vi "rsidr_core_global.vi"() -> ()   [LabVIEW 2020, in "Rohde&Schwarz RTx Oscilloscopes.lvlib"] (continued)
Options"="", "Flags"=0, "Help"="Searches for a subsystem bit of a status word.\n01X-string\n\nAvailable Repeated Capabilities:\nNone\n\nRemote-control command(s):\nSEARch:PROTocol:MILStd:STATus:SUBSystem"}, {"Level"=4, "Class Only"=FALSE, "Identifier"="RSRTX_ATTR_MILSTD_SEARCH_TERMINAL_BIT_STATUS", "Descriptive Name"="MILSTD Search Terminal Bit Status", "Data Type"=0, "Command"="SEAR:PROT:MILS:STAT:TERM", "Access"=2, "Range Table"="rsrtx_rngStatus", "Read Callback"="", "Write Callback"="", "Supported Models"="RTM|RTA", "Instrument Options"="", "Flags"=0, "Help"="Searches for a terminal bit of a status word.\n01X-string\n\nAvailable Repeated Capabilities:\nNone\n\nRemote-control command(s):\nSEARch:PROTocol:MILStd:STATus:TERMinal"}, {"Level"=3, "Class Only"=TRUE, "Identifier"="", "Descriptive Name"="Data", "Data Type"=0, "Command"="", "Access"=0, "Range Table"="", "Read Callback"="", "Write Callback"="", "Supported Models"="", "Instrument Options"="", "Flags"=0, "Help"="Searches for a data, that is specified."}, {"Level"=4, "Class Only"=FALSE, "Identifier"="RSRTX_ATTR_MILSTD_SEARCH_DATA_CONDITION", "Descriptive Name"="MILSTD Search Data Condition", "Data Type"=0, "Command"="SEAR:PROT:MILS:DATA:COND", "Access"=2, "Range Table"="rsrtx_rngMILSTDCondition", "Read Callback"="", "Write Callback"="", "Supported Models"="RTM|RTA", "Instrument Options"="", "Flags"=0, "Help"="For a data word, searches for a comparison condition.\n\nAvailable Repeated Capabilities:\nNone\n\nRemote-control command(s):\nSEARch:PROTocol:MILStd:DATA:CONDition"}, {"Level"=4, "Class Only"=FALSE, "Identifier"="RSRTX_ATTR_MILSTD_SEARCH_DATA_MINIMUM", "Descriptive Name"="MILSTD Search Data Minimum", "Data Type"=2, "Command"="SEAR:PROT:MILS:DATA:MIN", "Access"=2, "Range Table"="", "Read Callback"="", "Write Callback"="", "Supported Models"="RTM|RTA", "Instrument Options"="", "Flags"=0, "Help"="For a data word, searches for a minimum value.\n01X-string\n\nAvailable Repeated Capabilities:\nNone\n\nRemote-control command(s):\nSEARch:PROTocol:MILStd:DATA:MINimum"}, {"Level"=4, "Class Only"=FALSE, "Identifier"="RSRTX_ATTR_MILSTD_SEARCH_DATA_MAXIMUM", "Descriptive Name"="MILSTD Search Data Maximum", "Data Type"=2, "Command"="SEAR:PROT:MILS:DATA:MAX", "Access"=2, "Range Table"="", "Read Callback"="", "Write Callback"="", "Supported Models"="RTM|RTA", "Instrument Options"="", "Flags"=0, "Help"="For a data word, searches for a maximum value.\n01X-string\n\nAvailable Repeated Capabilities:\nNone\n\nRemote-control command(s):\nSEARch:PROTocol:MILStd:DATA:MAXimum"}, {"Level"=4, "Class Only"=FALSE, "Identifier"="RSRTX_ATTR_MILSTD_SEARCH_DATA_OFFSET", "Descriptive Name"="MILSTD Search Data Offset", "Data Type"=0, "Command"="SEAR:PROT:MILS:DATA:OFFS", "Access"=2, "Range Table"="", "Read Callback"="", "Write Callback"="", "Supported Models"="RTM|RTA", "Instrument Options"="", "Flags"=0, "Help"="For a data word, searches for a data offset.\n\nAvailable Repeated Capabilities:\nNone\n\nRemote-control command(s):\nSEARch:PROTocol:MILStd:DATA:OFFSet"}, {"Level"=4, "Class Only"=FALSE, "Identifier"="RSRTX_ATTR_MILSTD_SEARCH_DATA_OFFSET_WORDS", "Descriptive Name"="MILSTD Search Data Offset Words", "Data Type"=0, "Command"="SEAR:PROT:MILS:DATA:WORD", "Access"=2, "Range Table"="", "Read Callback"="", "Write Callback"="", "Supported Models"="RTM|RTA", "Instrument Options"="", "Flags"=0, "Help"="For a data word, searches for a number of words.\n\nAvailable Repeated Capabilities:\nNone\n\nRemote-control command(s):\nSEARch:PROTocol:MILStd:DATA:WORDs"}, {"Level"=2, "Class Only"=TRUE, "Identifier"="", "Descriptive Name"="ARINC 429", "Data Type"=0, "Command"="", "Access"=0, "Range Table"="", "Read Callback"="", "Write Callback"="", "Supported Models"="", "Instrument Options"="", "Flags"=0, "Help"="Configures ARINC 429 search settings."}, {"Level"=3, "Class Only"=FALSE, "Identifier"="RSRTX_ATTR_PROTOCOL_ARINC429_SEARCH_TYPE", "Descriptive Name"="Protocol ARINC429 Search Type", "Data Type"=0, "Command"="SEAR:PROT:ARIN:COND", "Access"=2, "Range Table"="rsrtx_rngARINC429Type", "Read Callback"="", "Write Callback"="", "Supported Models"="RTM|RTA", "Instrument Options"="", "Flags"=0, "Help"="Sets the event or combination of events to be searched for. Depending on the selected event, further settings are required.\n\nAvailable Repeated Capabilities:\nNone\n\nRemote-control command(s):\nSEARch:PROTocol:ARINc:CONDition"}, {"Level"=3, "Class Only"=FALSE, "Identifier"="RSRTX_ATTR_PROTOCOL_ARINC429_SEARCH_WORD_TYPE", "Descriptive Name"="Protocol ARINC429 Search Word Type", "Data Type"=0, "Command"="SEAR:PROT:ARIN:WORD", "Access"=2, "Range Table"="rsrtx_rngARINC429WordType", "Read Callback"="", "Write Callback"="", "Supported Models"="RTM|RTA", "Instrument Options"="", "Flags"=0, "Help"="Selects the word type to be searched for.\n\nAvailable Repeated Capabilities:\nNone\n\nRemote-control command(s):\nSEARch:PROTocol:ARINc:WORD[:TYPE]"}, {"Level"=3, "Class Only"=FALSE, "Identifier"="RSRTX_ATTR_PROTOCOL_ARINC429_SEARCH_ERROR", "Descriptive Name"="Protocol ARINC429 Search Error", "Data Type"=0, "Command"="SEAR:PROT:ARIN:ERR", "Access"=2, "Range Table"="rsrtx_rngARINC429Error", "Read Callback"="", "Write Callback"="", "Supported Models"="RTM|RTA", "Instrument Options"="", "Flags"=0, "Help"="Searches for an error condition.\n\nAvailable Repeated Capabilities:\nNone\n\nRemote-control command(s):\nSEARch:PROTocol:ARINc:ERRor"}, {"Level"=3, "Class Only"=TRUE, "Identifier"="", "Descriptive Name"="Label Data", "Data Type"=0, "Command"="", "Access"=0, "Range Table"="", "Read Callback"="", "Write Callback"="", "Supported Models"="", "Instrument Options"="", "Flags"=0, "Help"="Configures ARINC 429 search label+data settings."}, {"Level"=4, "Class Only"=FALSE, "Identifier"="RSRTX_ATTR_PROTOCOL_ARINC429_SEARCH_LABEL_PATTERN_CONDITION", "Descriptive Name"="Protocol ARINC429 Search Label Pattern Condition", "Data Type"=0, "Command"="SEAR:PROT:ARIN:LAB:COND", "Access"=2, "Range Table"="rsrtx_rngProtocolARINC429Operator", "Read Callback"="", "Write Callback"="", "Supported Models"="RTM|RTA", "Instrument Options"="", "Flags"=0, "Help"="Sets the comparison condition for label: If the pattern contains at least one X (don&apos;t care), you can trigger on values equal or not equal to the specified value. If the pattern contains only 0 and 1, you can also trigger on a range greater than or lower than the specified value.\n\nAvailable Repeated Capabilities:\nNone\n\nRemote-control command(s):\nSEARch:PROTocol:ARINc:LABel:CONDition"}, {"Level"=4, "Class Only"=FALSE, "Identifier"="RSRTX_ATTR_PROTOCOL_ARINC429_SEARCH_LABEL_PATTERN_MIN", "Descriptive Name"="Protocol ARINC429 Search Label Pattern Min", "Data Type"=2, "Command"="SEAR:PROT:ARIN:LAB:MIN", "Access"=2, "Range Table"="", "Read Callback"="", "Write Callback"="", "Supported Models"="RTM|RTA", "Instrument Options"="", "Flags"=0, "Help"="Searches for a minimum value of the label.\n\nAvailable Repeated Capabilities:\nNone\n\nRemote-control command(s):\nSEARch:PROTocol:ARINc:LABel:MINimum"}, {"Level"=4, "Class Only"=FALSE, "Identifier"="RSRTX_ATTR_PROTOCOL_ARINC429_SEARCH_LABEL_PATTERN_MAX", "Descriptive Name"="Protocol ARINC429 Search Label Pattern Max", "Data Type"=2, "Command"="SEAR:PROT:ARIN:LAB:MAX", "Access"=2, "Range Table"="", "Read Callback"="", "Write Callback"="", "Supported Models"="RTM|RTA", "Instrument Options"="", "Flags"=0, "Help"="Searches for a maximum value of the label if Label Pattern Condition is set to InRange or OutOfRange.\n\nAvailable Repeated Capabilities:\nNone\n\nRemote-control command(s):\nSEARch:PROTocol:ARINc:LABel:MAXimum"}, {"Level"=4, "Class Only"=FALSE, "Identifier"="RSRTX_ATTR_PROTOCOL_ARINC429_SEARCH_DATA_PATTERN_CONDITION", "Descriptive Name"="Protocol ARINC429 Search Data Pattern Condition", "Data Type"=0, "Command"="SEAR:PROT:ARIN:DATA:COND", "Access"=2, "Range Table"="rsrtx_rngProtocolARINC429Operator", "Read Callback"="", "Write Callback"="", "Supported Models"="RTM|RTA", "Instrument Options"="", "Flags"=0, "Help"="Sets the comparison condition for datal: If the pattern contains at least one X (don&apos;t care), you can trigger on values equal or not equal to the specified value. If the pattern contains only 0 and 1, you can also trigger on a range greater than or lower than the specified value.\n\nAvailable Repeated Capabilities:\nNone\n\nRemote-control command(s):\nSEARch:PROTocol:ARINc:DATA:CONDition"}, {"Level"=4, "Class Only"=FALSE, "Identifier"="RSRTX_ATTR_PROTOCOL_ARINC429_SEARCH_DATA_PATTERN_MIN", "Descriptive Name"="Protocol ARINC429 Search Data Pattern Min", "Data Type"=2, "Command"="SEAR:PROT:ARIN:DATA:MIN", "Access"=2, "Range Table"="", "Read Callback"="", "Write Callback"="", "Supported Models"="RTM|RTA", "Instrument Options"="", "Flags"=0, "Help"="Searches for a minimum value of the data.\n\nAvailable Repeated Capabilities:\nNone\n\nRemote-control command(s):\nSEARch:PROTocol:ARINc:DATA:MINimum"}, {"Level"=4, "Class Only"=FALSE, "Identifier"="RSRTX_ATTR_PROTOCOL_ARINC429_SEARCH_DATA_PATTERN_MAX", "Descriptive Name"="Protocol ARINC429 Search Data Pattern Max", "Data Type"=2, "Command"="SEAR:PROT:ARIN:DATA:MAX", "Access"=2, "Range Table"="", "Read Callback"="", "Write Callback"="", "Supported Models"="RTM|RTA", "Instrument Options"="", "Flags"=0, "Help"="Searches for a maximum value of the data  if Data Pattern Condition is set to InRange or OutOfRange.\n\nAvailable Repeated Capabilities:\nNone\n\nRemote-control command(s):\nSEARch:PROTocol:ARINc:DATA:MAX"}, {"Level"=4, "Class Only"=FALSE, "Identifier"="RSRTX_ATTR_PROTOCOL_ARINC429_SEARCH_DATA_OFFSET", "Descriptive Name"="Protocol ARINC429 Search Data Offset", "Data Type"=0, "Command"="SEAR:PROT:ARIN:DATA:OFFS", "Access"=2, "Range Table"="", "Read Callback"="", "Write Callback"="", "Supported Models"="RTM|RTA", "Instrument Options"="", "Flags"=0, "Help"="Searches for specified data offset.\n\nAvailable Repeated Capabilities:\nNone\n\nRemote-control command(s):\nSEARch:PROTocol:ARINc:DATA:OFFSet"}, {"Level"=4, "Class Only"=FALSE, "Identifier"="RSRTX_ATTR_PROTOCOL_ARINC429_SEARCH_DATA_SIZE", "Descriptive Name"="Protocol ARINC429 Search Data Size", "Data Type"=0, "Command"="SEAR:PROT:ARIN:DATA:SIZE", "Access"=2, "Range Table"="", "Read Callback"="", "Write Callback"="", "Supported Models"="RTM|RTA", "Instrument Options"="", "Flags"=0, "Help"="Searches for specified data size.\n\nAvailable Repeated Capabilities:\nNone\n\nRemote-control command(s):\nSEARch:PROTocol:ARINc:DATA:SIZE"}, {"Level"=4, "Class Only"=FALSE, "Identifier"="RSRTX_ATTR_PROTOCOL_ARINC429_SEARCH_DATA_FORMAT", "Descriptive Name"="Protocol ARINC429 Search Data Format", "Data Type"=0, "Command"="SEAR:PROT:ARIN:FORM", "Access"=2, "Range Table"="rsrtx_rngProtocolARINC429DataFormat", "Read Callback"="", "Write Callback"="", "Supported Models"="RTM|RTA", "Instrument Options"="", "Flags"=0, "Help"="Searches for a data format.\n\nAvailable Repeated Capabilities:\nNone\n\nRemote-control command(s):\nSEARch:PROTocol:ARINc:FORMat"}, {"Level"=4, "Class Only"=FALSE, "Identifier"="RSRTX_ATTR_PROTOCOL_ARINC429_SEARCH_SDI", "Descriptive Name"="Protocol ARINC429 Search SDI", "Data Type"=0, "Command"="SEAR:PROT:ARIN:SDI", "Access"=2, "Range Table"="rsrtx_rngARINCSsmSdi", "Read Callback"="", "Write Callback"="", "Supported Models"="RTM|RTA", "Instrument Options"="", "Flags"=0, "Help"="Searches for the specified source/destination identifier (SDI) bits.\n\nAvailable Repeated Capabilities:\nNone\n\nRemote-control command(s):\nSEARch:PROTocol:ARINc:SDI"}, {"Level"=4, "Class Only"=FALSE, "Identifier"="RSRTX_ATTR_PROTOCOL_ARINC429_SEARCH_SSM", "Descriptive Name"="Protocol ARINC429 Search SSM", "Data Type"=0, "Command"="SEAR:PROT:ARIN:SSM", "Access"=2, "Range Table"="rsrtx_rngARINCSsmSdi", "Read Callback"="", "Write Callback"="", "Supported Models"="RTM|RTA", "Instrument Options"="", "Flags"=0, "Help"="Searches for specified sign/status matrix (SSM) bits.\n\nAvailable Repeated Capabilities:\nNone\n\nRemote-control command(s):\nSEARch:PROTocol:ARINc:SSM"}, {"Level"=1, "Class Only"=TRUE, "Identifier"="", "Descriptive Name"="Protocols", "Data Type"=0, "Command"="", "Access"=0, "Range Table"="", "Read Callback"="", "Write Callback"="", "Supported Models"="", "Instrument Options"="", "Flags"=0, "Help"="Analyze serial protocols"}, {"Level"=2, "Class Only"=FALSE, "Identifier"="RSRTX_ATTR_PROTOCOL_ENABLED", "Descriptive Name"="Protocol Enabled", "Data Type"=3, "Command"="BUS{SerialBus}:STAT", "Access"=2, "Range Table"="", "Read Callback"="", "Write Callback"="", "Supported Models"="", "Instrument Options"="", "Flags"=0, "Help"="Switches the protocol display on or off.\n\nAvailable Repeated Capabilities:\nSerialBus: SB1, SB2, SB3, SB4\r\n\nRemote-control command(s):\nBUS<b>:STATe"}, {"Level"=2, "Class Only"=FALSE, "Identifier"="RSRTX_ATTR_PROTOCOL_TYPE", "Descriptive Name"="Protocol Type", "Data Type"=0, "Command"="BUS{SerialBus}:TYPE", "Access"=2, "Range Table"="rsrtx_rngProtocolType", "Read Callback"="", "Write Callback"="", "Supported Models"="", "Instrument Options"="", "Flags"=0, "Help"="Defines the bus or interface type for analysis. For most types, a special option to the instrument is required.\n\nAvailable Repeated Capabilities:\nSerialBus: SB1, SB2, SB3, SB4\r\n\nRemote-control command(s):\nBUS<b>:TYPE"}, {"Level"=2, "Class Only"=FALSE, "Identifier"="RSRTX_ATTR_BUS_SAVE_DECODED_DATA", "Descriptive Name"="Bus Save Decoded Data", "Data Type"=2, "Command"="BUS{SerialBus}:LIST:SAVE", "Access"=1, "Range Table"="", "Read Callback"="", "Write Callback"="", "Supported Models"="", "Instrument Options"="", "Flags"=0, "Help"="Saves the decoded data (frame table) to the specified CSV file (comma-separated list).\n\nAvailable Repeated Capabilities:\nSerialBus: SB1, SB2, SB3, SB4\r\n\nRemote-control command(s):\nBUS<b>:LIST:SAVE"}, {"Level"=2, "Class Only"=FALSE, "Identifier"="RSRTX_ATTR_PROTOCOL_CONTENT", "Descriptive Name"="Protocol Content", "Data Type"=2, "Command"="BUS{SerialBus}:LIST?", "Access"=0, "Range Table"="", "Read Callback"="", "Write Callback"="", "Supported Models"="", "Instrument Options"="", "Flags"=0, "Help"="Returns the contents of the frame table in block data format.\n\nAvailable Repeated Capabilities:\nSerialBus: SB1, SB2, SB3, SB4\r\n\nRemote-control command(s):\nBUS<b>:LIST?"}, {"Level"=2, "Class Only"=TRUE, "Identifier"="", "Descriptive Name"="Display", "Data Type"=0, "Command"="", "Access"=0, "Range Table"="", "Read Callback"="", "Write Callback"="", "Supported Models"="", "Instrument Options"="", "Flags"=0, "Help"="Display settings."}, {"Level"=3, "Class Only"=FALSE, "Identifier"="RSRTX_ATTR_PROTOCOL_DISPLAY_FORMAT", "Descriptive Name"="Protocol Display Format", "Data Type"=0, "Command"="BUS{SerialBus}:FORM", "Access"=2, "Range Table"="rsrtx_rngProtocolFormat", "Read Callback"="", "Write Callback"="", "Supported Models"="", "Instrument Options"="", "Flags"=0, "Help"="Sets the decoding format for the display on the screen.\n\nAvailable Repeated Capabilities:\nSerialBus: SB1, SB2, SB3, SB4\r\n\nRemote-control command(s):\nBUS<b>:FORMat"}, {"Level"=3, "Class Only"=FALSE, "Identifier"="RSRTX_ATTR_PROTOCOL_DISPLAY_HEIGHT", "Descriptive Name"="Protocol Display Height", "Data Type"=0, "Command"="BUS{SerialBus}:DSIZ", "Access"=2, "Range Table"="rsrtx_rngProtocolHeight", "Read Callback"="", "Write Callback"="", "Supported Models"="", "Instrument Options"="", "Flags"=0, "Help"="Sets the height of the decoded bus signal on the sreen.\n\nAvailable Repeated Capabilities:\nSerialBus: SB1, SB2, SB3, SB4\r\n\nRemote-control command(s):\nBUS<b>:DSIZe"}, {"Level"=3, "Class Only"=FALSE, "Identifier"="RSRTX_ATTR_PROTOCOL_DISPLAY_LINES", "Descriptive Name"="Protocol Display Lines", "Data Type"=3, "Command"="BUS{SerialBus}:DSIG", "Access"=2, "Range Table"="", "Read Callback"="", "Write Callback"="", "Supported Models"="", "Instrument Options"="", "Flags"=0, "Help"="Displays the individual bit lines above the decoded bus line.\n\nAvailable Repeated Capabilities:\nSerialBus: SB1, SB2, SB3, SB4\r\n\nRemote-control command(s):\nBUS<b>:DSIGnals"}, {"Level"=3, "Class Only"=FALSE, "Identifier"="RSRTX_ATTR_PROTOCOL_DISPLAY_VERTICAL", "Descriptive Name"="Protocol Display Vertical", "Data Type"=1, "Command"="BUS{SerialBus}:POS", "Access"=2, "Range Table"="rsrtx_rngProtocolVertical", "Read Callback"="", "Write Callback"="", "Supported Models"="", "Instrument Options"="", "Flags"=0, "Help"="Sets the vertical position of the decoded bus signal in divisions on the sreen.\n\nAvailable Repeated Capabilities:\nSerialBus: SB1, SB2, SB3, SB4\r\n\nRemote-control command(s):\nBUS<b>:POSition"}, {"Level"=3, "Class Only"=FALSE, "Identifier"="RSRTX_ATTR_PROTOCOL_DISPLAY_RESULTS", "Descriptive Name"="Protocol Display Results", "Data Type"=3, "Command"="BUS{SerialBus}:RES", "Access"=2, "Range Table"="", "Read Callback"="", "Write Callback"="", "Supported Models"="", "Instrument Options"="", "Flags"=0, "Help"="Displays or hides the table of decode results.\n\nAvailable Repeated Capabilities:\nSerialBus: SB1, SB2, SB3, SB4\r\n\nRemote-control command(s):\nBUS<b>:RESult"}, {"Level"=2, "Class Only"=TRUE, "Identifier"="", "Descriptive Name"="I2C", "Data Type"=0, "Command"="", "Access"=0, "Range Table"="", "Read Callback"="", "Write Callback"="", "Supported Models"="", "Instrument Options"="", "Flags"=0, "Help"="I2C (Inter-Integrated circuit bus) - decoding requires option R&S RTO-K1"}, {"Level"=3, "Class Only"=FALSE, "Identifier"="RSRTX_ATTR_PROTOCOL_I2C_CLOCK_SOURCE", "Descriptive Name"="Protocol I2C Clock Source", "Data Type"=0, "Command"="BUS{SerialBus}:I2C:CLOC:SOUR", "Access"=2, "Range Table"="RsRtx_rngChannelAndDigitalSource", "Read Callback"="", "Write Callback"="", "Supported Models"="", "Instrument Options"="", "Flags"=0, "Help"="Sets the waveform of the clock line.\n\nAvailable Repeated Capabilities:\nSerialBus: SB1, SB2, SB3, SB4\r\n\nRemote-control command(s):\nBUS<b>:I2C:CLOCk:SOURce"}, {"Level"=3, "Class Only"=FALSE, "Identifier"="RSRTX_ATTR_PROTOCOL_I2C_DATA_SOURCE", "Descriptive Name"="Protocol I2C Data Source", "Data Type"=0, "Command"="BUS{SerialBus}:I2C:DATA:SOUR", "Access"=2, "Range Table"="RsRtx_rngChannelAndDigitalSource", "Read Callback"="", "Write Callback"="", "Supported Models"="", "Instrument Options"="", "Flags"=0, "Help"="Sets the waveform of the data line.\n\nAvailable Repeated Capabilities:\nSerialBus: SB1, SB2, SB3, SB4\r\n\nRemote-control command(s):\nBUS<b>:I2C:DATA:SOURce"}, {"Level"=3, "Class Only"=FALSE, "Identifier"="RSRTX_ATTR_PROTOCOL_I2C_FRAME_COUNT", "Descriptive Name"="Protocol I2C Frame Count", "Data Type"=0, "Command"="BUS{SerialBus}:I2C:FCO?", "Access"=0, "Range Table"="", "Read Callback"="", "Write Callback"="", "Supported Models"="", "Instrument Options"="", "Flags"=0, "Help"="Queries the number of decoded frames.\n\nAvailable Repeated Capabilities:\nSerialBus: SB1, SB2, SB3, SB4\r\n\nRemote-control command(s):\nBUS<b>:I2C:FCOunt?"}, {"Level"=3, "Class Only"=FALSE, "Identifier"="RSRTX_ATTR_PROTOCOL_I2C_SELECTED_FRAME", "Descriptive Name"="Protocol I2C Selected Frame", "Data Type"=0, "Command"="", "Access"=2, "Range Table"="", "Read Callback"="", "Write Callback"="", "Supported Models"="", "Instrument Options"="", "Flags"=0, "Help"="Sets selector repeated capability Frame.\n\nAvailable Repeated Capabilities:\nNone\n\nRemote-control command(s):\n"}, {"Level"=3, "Class Only"=FALSE, "Identifier"="RSRTX_ATTR_PROTOCOL_I2C_FRAME_DATA", "Descriptive Name"="Protocol I2C Frame Data", "Data Type"=2, "Command"="BUS{SerialBus}:I2C:FRAM<Frame>:DATA?", "Access"=0, "Range Table"="", "Read Callback"="rsrtx_FormatI2CFrameRepCapString_ReadCallback.vi", "Write Callback"="", "Supported Models"="", "Instrument Options"="", "Flags"=0, "Help"="Returns the data words of the specified frame.\n\nAvailable Repeated Capabilities:\nSerialBus: SB1, SB2, SB3, SB4\r\n\nRemote-control command(s):\nBUS<b>:I2C:FRAMe<n>:DATA?"}, {"Level"=3, "Class Only"=FALSE, "Identifier"="RSRTX_ATTR_PROTOCOL_I2C_FRAME_STATUS", "Descriptive Name"="Protocol I2C Frame Status", "Data Type"=0, "Command"="BUS{SerialBus}:I2C:FRAM<Frame>:STAT?", "Access"=0, "Range Table"="rsrtx_rngProtocolI2CFrameState", "Read Callback"="rsrtx_FormatI2CFrameRepCapInt_ReadCallback.vi", "Write Callback"="", "Supported Models"="", "Instrument Options"="", "Flags"=0, "Help"="Returns the overall state of the frame.\n\nAvailable Repeated Capabilities:\nSerialBus: SB1, SB2, SB3, SB4\r\n\nRemote-control command(s):\nBUS<b>:I2C:FRAMe<n>:STATus?"}, {"Level"=3, "Class Only"=FALSE, "Identifier"="RSRTX_ATTR_PROTOCOL_I2C_FRAME_START", "Descriptive Name"="Protocol I2C Frame Start", "Data Type"=1, "Command"="BUS{SerialBus}:I2C:FRAM<Frame>:STAR?", "Access"=0, "Range Table"="", "Read Callback"="rsrtx_FormatI2CFrameRepCapReal_ReadCallback.vi", "Write Callback"="", "Supported Models"="", "Instrument Options"="", "Flags"=0, "Help"="Returns the start time of the specified frame.\n\nAvailable Repeated Capabilities:\nSerialBus: SB1, SB2, SB3, SB4\r\n\nRemote-control command(s):\nBUS<b>:I2C:FRAMe<n>:STARt?"}, {"Level"=3, "Class Only"=FALSE, "Identifier"="RSRTX_ATTR_PROTOCOL_I2C_FRAME_END", "Descriptive Name"="Protocol I2C Frame End", "Data Type"=1, "Command"="BUS{SerialBus}:I2C:FRAM<Frame>:STOP?", "Access"=0, "Range Table"="", "Read Callback"="rsrtx_FormatI2CFrameRepCapReal_ReadCallback.vi", "Write Callback"="", "Supported Models"="", "Instrument Options"="", "Flags"=0, "Help"="Returns the end time of the specified frame.\n\nAvailable Repeated Capabilities:\nSerialBus: SB1, SB2, SB3, SB4\r\n\nRemote-control command(s):\nBUS<b>:I2C:FRAMe<n>:STOP?"}, {"Level"=3, "Class Only"=FALSE, "Identifier"="RSRTX_ATTR_PROTOCOL_I2C_FRAME_TRANSFER_DIRECTION", "Descriptive Name"="Protocol I2C Frame Transfer Direction", "Data Type"=0, "Command"="BUS{SerialBus}:I2C:FRAM<Frame>:ACC?", "Access"=0, "Range Table"="rsrtx_rngI2CFrameTransferDirection", "Read Callback"="rsrtx_FormatI2CFrameRepCapInt_ReadCallback.vi", "Write Callback"="", "Supported Models"="", "Instrument Options"="", "Flags"=0, "Help"="Returns the transfer direction - read or write access from master to slave.\n\nAvailable Repeated Capabilities:\nSerialBus: SB1, SB2, SB3, SB4\r\n\nRemote-control command(s):\nBUS<b>:I2C:FRAMe<n>:ACCess?"}, {"Level"=3, "Class Only"=FALSE, "Identifier"="RSRTX_ATTR_PROTOCOL_I2C_FRAME_ADDRESS_ACKNOWLEDGE", "Descriptive Name"="Protocol I2C Frame Address Acknowledge", "Data Type"=0, "Command"="BUS{SerialBus}:I2C:FRAM<Frame>:AACC?", "Access"=0, "Range Table"="rsrtx_rngProtocolAckBit", "Read Callback"="rsrtx_FormatI2CFrameRepCapInt_ReadCallback.vi", "Write Callback"="", "Supported Models"="", "Instrument Options"="", "Flags"=0, "Help"="Returns the address acknowledge bit value for the indicated frame.\n\nAvailable Repeated Capabilities:\nSerialBus: SB1, SB2, SB3, SB4\r\n\nRemote-control command(s):\nBUS<b>:I2C:FRAMe<n>:AACCess?"}, {"Level"=3, "Class Only"=FALSE, "Identifier"="RSRTX_ATTR_PROTOCOL_I2C_FRAME_ADDRESS_ENABLED", "Descriptive Name"="Protocol I2C Frame Address Enabled", "Data Type"=3, "Command"="BUS{SerialBus}:I2C:FRAM<Frame>:ACOM?", "Access"=0, "Range Table"="", "Read Callback"="rsrtx_FormatI2CFrameRepCapBool_ReadCallback.vi", "Write Callback"="", "Supported Models"="", "Instrument Options"="", "Flags"=0, "Help"="Returns the state of the address.\n\nAvailable Repeated Capabilities:\nSerialBus: SB1, SB2, SB3, SB4\r\n\nRemote-control command(s):\nBUS<b>:I2C:FRAMe<n>:ACOMplete?"}, {"Level"=3, "Class Only"=FALSE, "Identifier"="RSRTX_ATTR_PROTOCOL_I2C_FRAME_ADDRESS_START_ACK_BIT", "Descriptive Name"="Protocol I2C Frame Address Start Ack Bit", "Data Type"=1, "Command"="BUS{SerialBus}:I2C:FRAM<Frame>:ADBS?", "Access"=0, "Range Table"="", "Read Callback"="rsrtx_FormatI2CFrameRepCapReal_ReadCallback.vi", "Write Callback"="", "Supported Models"="", "Instrument Options"="", "Flags"=0, "Help"="Returns the start time of the address acknowledge bit.\n\nAvailable Repeated Capabilities:\nSerialBus: SB1, SB2, SB3, SB4\r\n\nRemote-control command(s):\nBUS<b>:I2C:FRAMe<n>:ADBStart?"}, {"Level"=3, "Class Only"=FALSE, "Identifier"="RSRTX_ATTR_PROTOCOL_I2C_FRAME_ADDRESS", "Descriptive Name"="Protocol I2C Frame Address", "Data Type"=0, "Command"="BUS{SerialBus}:I2C:FRAM<Frame>:ADDR?", "Access"=0, "Range Table"="", "Read Callback"="rsrtx_FormatI2CFrameRepCapInt_ReadCallback.vi", "Write Callback"="", "Supported Models"="", "Instrument Options"="", "Flags"=0, "Help"="Returns the decimal address value of the indicated frame including the R/W bit.\n\nAvailable Repeated Capabilities:\nSerialBus: SB1, SB2, SB3, SB4\r\n\nRemote-control command(s):\nBUS<b>:I2C:FRAMe<n>:ADDRess?"}, {"Level"=3, "Class Only"=FALSE, "Identifier"="RSRTX_ATTR_PROTOCOL_I2C_FRAME_ADDRESS_WITHOUT_BIT", "Descriptive Name"="Protocol I2C Frame Address Without Bit", "Data Type"=0, "Command"="BUS{SerialBus}:I2C:FRAM<Frame>:ADEV?", "Access"=0, "Range Table"="", "Read Callback"="rsrtx_FormatI2CFrameRepCapInt_ReadCallback.vi", "Write Callback"="", "Supported Models"="", "Instrument Options"="", "Flags"=0, "Help"="Returns the decimal address value of the indicated frame without R/W bit.\n\nAvailable Repeated Capabilities:\nSerialBus: SB1, SB2, SB3, SB4\r\n\nRemote-control command(s):\nBUS<b>:I2C:FRAMe<n>:ADEVice?"}, {"Level"=3, "Class Only"=FALSE, "Identifier"="RSRTX_ATTR_PROTOCOL_I2C_FRAME_ADDRESS_LENGTH", "Descriptive Name"="Protocol I2C Frame Address Length", "Data Type"=0, "Command"="BUS{SerialBus}:I2C:FRAM<Frame>:AMOD?", "Access"=0, "Range Table"="rsrtx_rngFrameAddressLength", "Read Callback"="rsrtx_FormatI2CFrameRepCapInt_ReadCallback.vi", "Write Callback"="", "Supported Models"="", "Instrument Options"="", "Flags"=0, "Help"="Returns the address length.\n\nAvailable Repeated Capabilities:\nSerialBus: SB1, SB2, SB3, SB4\r\n\nRemote-control command(s):\nBUS<b>:I2C:FRAMe<n>:AMODe?"}, {"Level"=3, "Class Only"=FALSE, "Identifier"="RSRTX_ATTR_PROTOCOL_I2C_FRAME_ADDRESS_START", "Descriptive Name"="Protocol I2C Frame Address Start", "Data Type"=1, "Command"="BUS{SerialBus}:I2C:FRAM<Frame>:AST?", "Access"=0, "Range Table"="", "Read Callback"="rsrtx_FormatI2CFrameRepCapReal_ReadCallback.vi", "Write Callback"="", "Supported Models"="", "Instrument Options"="", "Flags"=0, "Help"="Returns the start time of the address for the indicated frame.\n\nAvailable Repeated Capabilities:\nSerialBus: SB1, SB2, SB3, SB4\r\n\nRemote-control command(s):\nBUS<b>:I2C:FRAMe<n>:ASTart?"}, {"Level"=3, "Class Only"=FALSE, "Identifier"="RSRTX_ATTR_PROTOCOL_I2C_SELECTED_BYTE", "Descriptive Name"="Protocol I2C Selected Byte", "Data Type"=0, "Command"="", "Access"=2, "Range Table"="", "Read Callback"="", "Write Callback"="", "Supported Models"="", "Instrument Options"="", "Flags"=0, "Help"="Sets selector repeated capability Byte.\n\nAvailable Repeated Capabilities:\nNone\n\nRemote-control command(s):\n"}, {"Level"=3, "Class Only"=FALSE, "Identifier"="RSRTX_ATTR_PROTOCOL_I2C_BYTE_COUNT", "Descriptive Name"="Protocol I2C Byte Count", "Data Type"=0, "Command"="BUS{SerialBus}:I2C:FRAM<Frame>:BCO?", "Access"=0, "Range Table"="", "Read Callback"="rsrtx_FormatI2CFrameRepCapInt_ReadCallback.vi", "Write Callback"="", "Supported Models"="", "Instrument Options"="", "Flags"=0, "Help"="Returns the number of data bytes in the specified frame.\n\nAvailable Repeated Capabilities:\nSerialBus: SB1, SB2, SB3, SB4\r\n\nRemote-control command(s):\nBUS<b>:I2C:FRAMe<n>:BCOunt?"}, {"Level"=3, "Class Only"=FALSE, "Identifier"="RSRTX_ATTR_PROTOCOL_I2C_BYTE_ACK_BIT", "Descriptive Name"="Protocol I2C Byte Ack Bit", "Data Type"=0, "Command"="BUS{SerialBus}:I2C:FRAM<Frame>:BYTE<Byte>:ACC?", "Access"=0, "Range Table"="rsrtx_rngProtocolAckBit", "Read Callback"="rsrtx_FormatI2CFrameByteRepCapInt_ReadCallback.vi", "Write Callback"="", "Supported Models"="", "Instrument Options"="", "Flags"=0, "Help"="Returns the acknowledge bit value of the specified data byte.\n\nAvailable Repeated Capabilities:\nSerialBus: SB1, SB2, SB3, SB4\r\n\nRemote-control command(s):\nBUS<b>:I2C:FRAMe<n>:BYTE<o>:ACCess?"}, {"Level"=3, "Class Only"=FALSE, "Identifier"="RSRTX_ATTR_PROTOCOL_I2C_BYTE_ACK_BIT_START", "Descriptive Name"="Protocol I2C Byte Ack Bit Start", "Data Type"=1, "Command"="BUS{SerialBus}:I2C:FRAM<Frame>:BYTE<Byte>:ACKS?", "Access"=0, "Range Table"="", "Read Callback"="rsrtx_FormatI2CFrameByteRepCapReal_ReadCallback.vi", "Write Callback"="", "Supported Models"="", "Instrument Options"="", "Flags"=0, "Help"="Returns the start time of the acknowledge bit of the specified byte.\n\nAvailable Repeated Capabilities:\nSerialBus: SB1, SB2, SB3, SB4\r\n\nRemote-control command(s):\nBUS<b>:I2C:FRAMe<n>:BYTE<o>:ACKStart?"}, {"Level"=3, "Class Only"=FALSE, "Identifier"="RSRTX_ATTR_PROTOCOL_I2C_BYTE_ENABLED", "Descriptive Name"="Protocol I2C Byte Enabled", "Data Type"=3, "Command"="BUS{SerialBus}:I2C:FRAM<Frame>:BYTE<Byte>:COMP?", "Access"=0, "Range Table"="", "Read Callback"="rsrtx_FormatI2CFrameByteRepCapBool_ReadCallback.vi", "Write Callback"="", "Supported Models"="", "Instrument Options"="", "Flags"=0, "Help"="Returns the state of the byte.\n\nAvailable Repeated Capabilities:\nSerialBus: SB1, SB2, SB3, SB4\r\n\nRemote-control command(s):\nBUS<b>:I2C:FRAMe<n>:BYTE<o>:COMPlete?"}, {"Level"=3, "Class Only"=FALSE, "Identifier"="RSRTX_ATTR_PROTOCOL_I2C_BYTE_START", "Descriptive Name"="Protocol I2C Byte Start", "Data Type"=1, "Command"="BUS{SerialBus}:I2C:FRAM<Frame>:BYTE<Byte>:STAR?", "Access"=0, "Range Table"="", "Read Callback"="rsrtx_FormatI2CFrameByteRepCapReal_ReadCallback.vi", "Write Callback"="", "Supported Models"="", "Instrument Options"="", "Flags"=0, "Help"="Returns the start time of the specified data byte.\n\nAvailable Repeated Capabilities:\nSerialBus: SB1, SB2, SB3, SB4\r\n\nRemote-control command(s):\nBUS<b>:I2C:FRAMe<n>:BYTE<o>:STARt?"}, {"Level"=3, "Class Only"=FALSE, "Identifier"="RSRTX_ATTR_PROTOCOL_I2C_BYTE_VALUE", "Descriptive Name"="Protocol I2C Byte Value", "Data Type"=0, "Command"="BUS{SerialBus}:I2C:FRAM<Frame>:BYTE<Byte>:VAL?", "Access"=0, "Range Table"="", "Read Callback"="rsrtx_FormatI2CFrameByteRepCapInt_ReadCallback.vi", "Write Callback"="", "Supported Models"="", "Instrument Options"="", "Flags"=0, "Help"="Returns the decimal value of the specified byte.\n\nAvailable Repeated Capabilities:\nSerialBus: SB1, SB2, SB3, SB4\r\n\nRemote-control command(s):\nBUS<b>:I2C:FRAMe<n>:BYTE<o>:VALue?"}, {"Level"=2, "Class Only"=TRUE, "Identifier"="", "Descriptive Name"="SPI", "Data Type"=0, "Command"="", "Access"=0, "Range Table"="", "Read Callback"="", "Write Callback"="", "Supported Models"="", "Instrument Options"="", "Flags"=0, "Help"="SPI (Serial Peripheral Interface) - decoding requires option R&S RTO-K1"}, {"Level"=3, "Class Only"=FALSE, "Identifier"="RSRTX_ATTR_PROTOCOL_SPI_CLOCK_SOURCE", "Descriptive Name"="Protocol SPI Clock Source", "Data Type"=0, "Command"="BUS{SerialBus}:SPI:CLOC:SOUR", "Access"=2, "Range Table"="RsRtx_rngChannelAndDigitalSource", "Read Callback"="", "Write Callback"="", "Supported Models"="", "Instrument Options"="", "Flags"=0, "Help"="Sets the input channel for the clock lines.\n\nAvailable Repeated Capabilities:\nSerialBus: SB1, SB2, SB3, SB4\r\n\nRemote-control command(s):\nBUS<b>:SPI:CLOCk:SOURce"}, {"Level"=3, "Class Only"=FALSE, "Identifier"="RSRTX_ATTR_PROTOCOL_SPI_DATA_SOURCE", "Descriptive Name"="Protocol SPI Data Source", "Data Type"=0, "Command"="BUS{SerialBus}:SPI:DATA:SOUR", "Access"=2, "Range Table"="rsrtx_rngMOSISource", "Read Callback"="", "Write Callback"="", "Supported Models"="", "Instrument Options"="", "Flags"=0, "Help"="Sets the input channel for the data lines.\n\nAvailable Repeated Capabilities:\nSerialBus: SB1, SB2, SB3, SB4\r\n\nRemote-control command(s):\nBUS<b>:SPI:DATA:SOURce"}, {"Level"=3, "Class Only"=FALSE, "Identifier"="RSRTX_ATTR_PROTOCOL_SPI_MOSI_SOURCE", "Descriptive Name"="Protocol SPI MOSI Source", "Data Type"=0, "Command"="BUS{SerialBus}:SPI:MOSI:SOUR", "Access"=2, "Range Table"="rsrtx_rngMOSISource", "Read Callback"="", "Write Callback"="", "Supported Models"="", "Instrument Options"="", "Flags"=0, "Help"="Selects the input channel of the MOSI line.\n\nAvailable Repeated Capabilities:\nSerialBus: SB1, SB2, SB3, SB4\r\n\nRemote-control command(s):\nBUS<b>:SPI:MOSI:SOURce"}, {"Level"=3, "Class Only"=FALSE, "Identifier"="RSRTX_ATTR_PROTOCOL_SPI_MISO_SOURCE", "Descriptive Name"="Protocol SPI MISO Source", "Data Type"=0, "Command"="BUS{SerialBus}:SPI:MISO:SOUR", "Access"=2, "Range Table"="rsrtx_rngMISOSource", "Read Callback"="", "Write Callback"="", "Supported Models"="", "Instrument Options"="", "Flags"=0, "Help"="Selects the input channel of the optional MISO line.\n\nAvailable Repeated Capabilities:\nSerialBus: SB1, SB2, SB3, SB4\r\n\nRemote-control command(s):\nBUS<b>:SPI:MISO:SOURce"}, {"Level"=3, "Class Only"=FALSE, "Identifier"="RSRTX_ATTR_PROTOCOL_SPI_CLOCK_POLARITY", "Descriptive Name"="Protocol SPI Clock Polarity", "Data Type"=0, "Command"="BUS{SerialBus}:SPI:CLOC:POL", "Access"=2, "Range Table"="rsrtx_rngProtocolSPIPolarity", "Read Callback"="", "Write Callback"="", "Supported Models"="", "Instrument Options"="", "Flags"=0, "Help"="Selects whether transmitted signal is high active (high = 1) or low active (low= 1).\n\nAvailable Repeated Capabilities:\nSerialBus: SB1, SB2, SB3, SB4\r\n\nRemote-control command(s):\nBUS<b>:SPI:CLOCk:POLarity"}, {"Level"=3, "Class Only"=FALSE, "Identifier"="RSRTX_ATTR_PROTOCOL_SPI_CS_POLARITY", "Descriptive Name"="Protocol SPI CS Polarity", "Data Type"=0, "Command"="BUS{SerialBus}:SPI:CS:POL", "Access"=2, "Range Table"="rsrtx_rngProtocolSPIPolarity", "Read Callback"="", "Write Callback"="", "Supported Models"="", "Instrument Options"="", "Flags"=0, "Help"="Selects wether the chip select signal is high active (high = 1) or low active (low = 1).\n\nAvailable Repeated Capabilities:\nSerialBus: SB1, SB2, SB3, SB4\r\n\nRemote-control command(s):\nBUS<b>:SPI:CS:POLarity"}, {"Level"=3, "Class Only"=FALSE, "Identifier"="RSRTX_ATTR_PROTOCOL_SPI_CS_SOURCE", "Descriptive Name"="Protocol SPI CS Source", "Data Type"=0, "Command"="BUS{SerialBus}:SPI:CS:SOUR", "Access"=2, "Range Table"="rsrtx_rngSPIChipSelectSource", "Read Callback"="", "Write Callback"="", "Supported Models"="", "Instrument Options"="", "Flags"=0, "Help"="Selects the input channel of the chip select line.\n\nAvailable Repeated Capabilities:\nSerialBus: SB1, SB2, SB3, SB4\r\n\nRemote-control command(s):\nBUS<b>:SPI:CS:SOURce"}, {"Level"=3, "Class Only"=FALSE, "Identifier"="RSRTX_ATTR_PROTOCOL_SPI_DATA_POLARITY", "Descriptive Name"="Protocol SPI Data Polarity", "Data Type"=0, "Command"="BUS{SerialBus}:SPI:DATA:POL", "Access"=2, "Range Table"="rsrtx_rngProtocolSPIPolarity", "Read Callback"="", "Write Callback"="", "Supported Models"="", "Instrument Options"="", "Flags"=0, "Help"="Selects whether transmitted signal is high active (high = 1) or low active (low= 1).\n\nAvailable Repeated Capabilities:\nSerialBus: SB1, SB2, SB3, SB4\r\n\nRemote-control command(s):\nBUS<b>:SPI:DATA:POLarity"}, {"Level"=3, "Class Only"=FALSE, "Identifier"="RSRTX_ATTR_PROTOCOL_SPI_BIT_ORDER", "Descriptive Name"="Protocol SPI Bit Order", "Data Type"=0, "Command"="BUS{SerialBus}:SPI:BORD", "Access"=2, "Range Table"="rsrtx_rngProtocolSPIBitOrder", "Read Callback"="", "Write Callback"="", "Supported Models"="", "Instrument Options"="", "Flags"=0, "Help"="Defines if the data of the messages starts with msb (most significant bit) or lsb (least significant bit).\n\nAvailable Repeated Capabilities:\nSerialBus: SB1, SB2, SB3, SB4\r\n\nRemote-control command(s):\nBUS<b>:SPI:BORDer"}, {"Level"=3, "Class Only"=FALSE, "Identifier"="RSRTX_ATTR_PROTOCOL_SPI_WORD_LENGTH", "Descriptive Name"="Protocol SPI Word Length", "Data Type"=0, "Command"="BUS{SerialBus}:SPI:SSIZ", "Access"=2, "Range Table"="rsrtx_rngProtocolSPIWordLength", "Read Callback"="", "Write Callback"="", "Supported Models"="", "Instrument Options"="", "Flags"=0, "Help"="Sets the number of bits in a message.\n\nAvailable Repeated Capabilities:\nSerialBus: SB1, SB2, SB3, SB4\r\n\nRemote-control command(s):\nBUS<b>:SPI:SSIZe"}, {"Level"=3, "Class Only"=FALSE, "Identifier"="RSRTX_ATTR_PROTOCOL_SPI_MOSI_POLARITY", "Descriptive Name"="Protocol SPI MOSI Polarity", "Data Type"=0, "Command"="BUS{SerialBus}:SPI:MOSI:POL", "Access"=2, "Range Table"="rsrtx_rngProtocolSPIMISOPolarity", "Read Callback"="", "Write Callback"="", "Supported Models"="", "Instrument Options"="", "Flags"=0, "Help"="Selects if transmitted data is high active (high = 1) or low active (low = 1) on the MOSI/MISO line.\n\nAvailable Repeated Capabilities:\nSerialBus: SB1, SB2, SB3, SB4\r\n\nRemote-control command(s):\nBUS<b>:SPI:MOSI:POLarity"}, {"Level"=3, "Class Only"=FALSE, "Identifier"="RSRTX_ATTR_PROTOCOL_SPI_MISO_POLARITY", "Descriptive Name"="Protocol SPI MISO Polarity", "Data Type"=0, "Command"="BUS{SerialBus}:SPI:MISO:POL", "Access"=2, "Range Table"="rsrtx_rngProtocolSPIMISOPolarity", "Read Callback"="", "Write Callback"="", "Supported Models"="", "Instrument Options"="", "Flags"=0, "Help"="Selects whether transmitted data is high active (high = 1) or low active (low = 1) on the MISO line.\n\nAvailable Repeated Capabilities:\nSerialBus: SB1, SB2, SB3, SB4\r\n\nRemote-control command(s):\nBUS<b>:SPI:MISO:POLarity"}, {"Level"=3, "Class Only"=FALSE, "Identifier"="RSRTX_ATTR_PROTOCOL_SPI_FRAME_COUNT", "Descriptive Name"="Protocol SPI Frame Count", "Data Type"=0, "Command"="BUS{SerialBus}:SPI:FCO?", "Access"=0, "Range Table"="", "Read Callback"="", "Write Callback"="", "Supported Models"="", "Instrument Options"="", "Flags"=0, "Help"="Queries the number of decoded frames.\n\nAvailable Repeated Capabilities:\nSerialBus: SB1, SB2, SB3, SB4\r\n\nRemote-control command(s):\nBUS<b>:SPI:FCOunt?"}, {"Level"=3, "Class Only"=FALSE, "Identifier"="RSRTX_ATTR_PROTOCOL_SPI_SELECTED_FRAME", "Descriptive Name"="Protocol SPI Selected Frame", "Data Type"=0, "Command"="", "Access"=2, "Range Table"="", "Read Callback"="", "Write Callback"="", "Supported Models"="", "Instrument Options"="", "Flags"=0, "Help"="Sets selector repeated capability Frame.\n\nAvailable Repeated Capabilities:\nNone\n\nRemote-control command(s):\n"}, {"Level"=3, "Class Only"=FALSE, "Identifier"="RSRTX_ATTR_PROTOCOL_SPI_FRAME_STATUS", "Descriptive Name"="Protocol SPI Frame Status", "Data Type"=0, "Command"="BUS{SerialBus}:SPI:FRAM<Frame>:STAT?", "Access"=0, "Range Table"="rsrtx_rngProtocolSPIFrameState", "Read Callback"="rsrtx_FormatSPIFrameRepCapInt_ReadCallback.vi", "Write Callback"="", "Supported Models"="", "Instrument Options"="", "Flags"=0, "Help"="Returns the overall state of the specified frame.\n\nAvailable Repeated Capabilities:\nSerialBus: SB1, SB2, SB3, SB4\r\n\nRemote-control command(s):\nBUS<b>:SPI:FRAMe<n>:STATus?"}, {"Level"=3, "Class Only"=FALSE, "Identifier"="RSRTX_ATTR_PROTOCOL_SPI_FRAME_START", "Descriptive Name"="Protocol SPI Frame Start", "Data Type"=1, "Command"="BUS{SerialBus}:SPI:FRAM<Frame>:STARt?", "Access"=0, "Range Table"="", "Read Callback"="rsrtx_FormatSPIFrameRepCapReal_ReadCallback.vi", "Write Callback"="", "Supported Models"="", "Instrument Options"="", "Flags"=0, "Help"="Returns the start time of the specified frame.\n\nAvailable Repeated Capabilities:\nSerialBus: SB1, SB2, SB3, SB4\r\n\nRemote-control command(s):\nBUS<b>:SPI:FRAMe<n>:STARt?"}, {"Level"=3, "Class Only"=FALSE, "Identifier"="RSRTX_ATTR_PROTOCOL_SPI_FRAME_END", "Descriptive Name"="Protocol SPI Frame End", "Data Type"=1, "Command"="BUS{SerialBus}:SPI:FRAM<Frame>:STOP?", "Access"=0, "Range Table"="", "Read Callback"="rsrtx_FormatSPIFrameRepCapReal_ReadCallback.vi", "Write Callback"="", "Supported Models"="", "Instrument Options"="", "Flags"=0, "Help"="Returns the end time of the specified frame.\n\nAvailable Repeated Capabilities:\nSerialBus: SB1, SB2, SB3, SB4\r\n\nRemote-control command(s):\nBUS<b>:SPI:FRAMe<n>:STOP?"}, {"Level"=3, "Class Only"=FALSE, "Identifier"="RSRTX_ATTR_PROTOCOL_SPI_FRAME_DATA_MOSI", 
